vi "logForceActuatorInfo.vi"(8 "error in (no error)":errorcluster, 10 "EventForceActuatorInfo":T1, 11 "M1M3SAL in":refnum<class "M1M3SAL.lvclass">) -> (0 "error out":errorcluster, 3 "M1M3SAL out":refnum<class "M1M3SAL.lvclass">)   [LabVIEW 2016, in "M1M3SupportCommunicator.lvlib" / "M1M3SAL.lvclass"]
uses:
  M1M3SAL.lvclass
  DataTypes/Topics/EventForceActuatorInfo.ctl
  DataTypes/Topics/Parts/Timestamp.ctl
  DataTypes/MessageHeader.ctl
  DataTypes/MessageTypes.ctl
  DataTypes/MessageTopics.ctl
  M1M3SAL.lvclass/M1M3SAL.ctl
  writeU8.vi
  writeSGL.vi
  writeI64.vi
  writeBoolean.vi
  M1M3SupportCommunicator.lvlib
  DataTypes/Topics/M1M3SupportTopics.lvlib
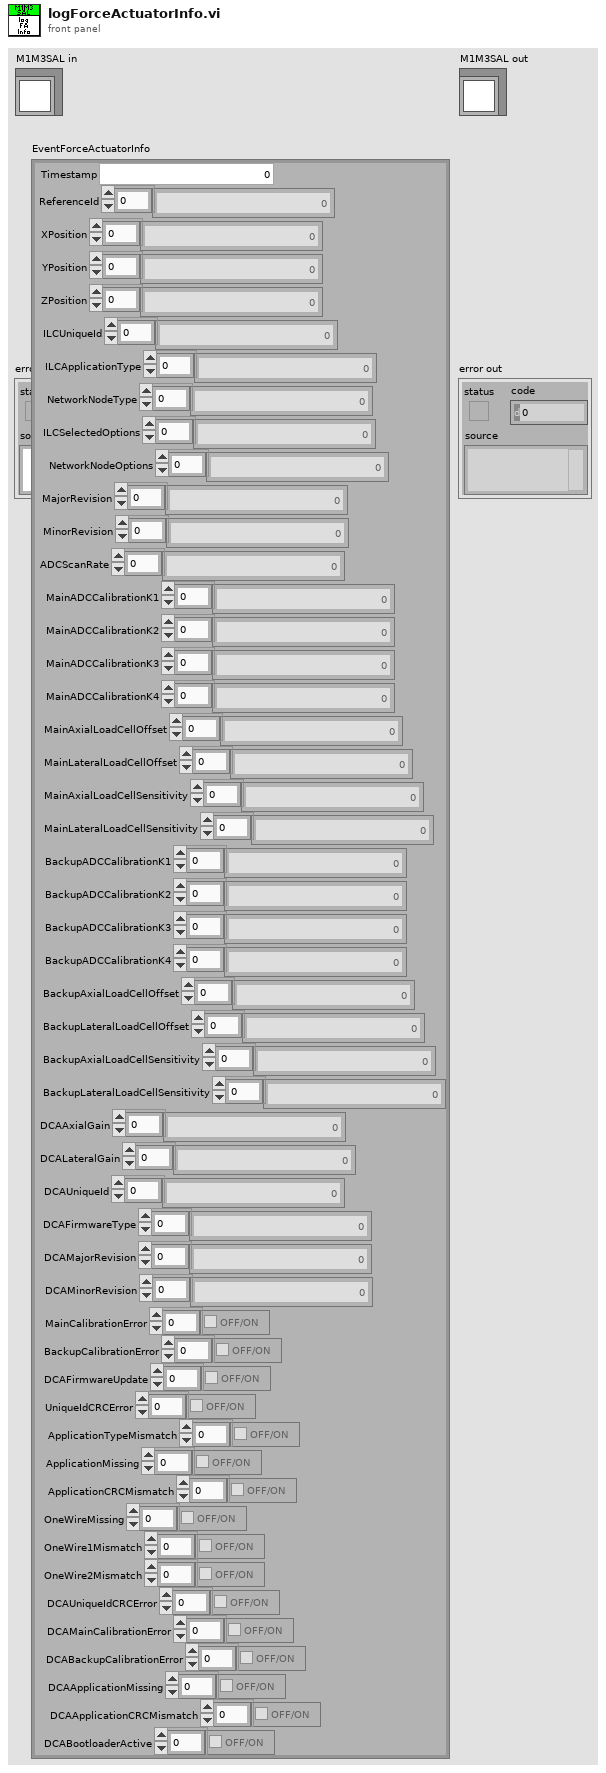
[diagram p1: front panel]
types:
  T1 = typedef "M1M3SupportTopics.lvlib/EventForceActuatorInfo.ctl" = cluster{"Timestamp":T2, "ReferenceId":i32[], "XPosition":sgl[], "YPosition":sgl[], "ZPosition":sgl[], "ILCUniqueId":i64[], "ILCApplicationType":u8[], "NetworkNodeType":u8[], "ILCSelectedOptions":u8[], "NetworkNodeOptions":u8[], "MajorRevision":u8[], "MinorRevision":u8[], "ADCScanRate":u8[], "MainADCCalibrationK1":sgl[], "MainADCCalibrationK2":sgl[], "MainADCCalibrationK3":sgl[], "MainADCCalibrationK4":sgl[], "MainAxialLoadCellOffset":sgl[], "MainLateralLoadCellOffset":sgl[], "MainAxialLoadCellSensitivity":sgl[], "MainLateralLoadCellSensitivity":sgl[], "BackupADCCalibrationK1":sgl[], "BackupADCCalibrationK2":sgl[], "BackupADCCalibrationK3":sgl[], "BackupADCCalibrationK4":sgl[], "BackupAxialLoadCellOffset":sgl[], "BackupLateralLoadCellOffset":sgl[], "BackupAxialLoadCellSensitivity":sgl[], "BackupLateralLoadCellSensitivity":sgl[], "DCAAxialGain":sgl[], "DCALateralGain":sgl[], "DCAUniqueId":i64[], "DCAFirmwareType":u8[], "DCAMajorRevision":u8[], "DCAMinorRevision":u8[], "MainCalibrationError":bool[], "BackupCalibrationError":bool[], "DCAFirmwareUpdate":bool[], "UniqueIdCRCError":bool[], "ApplicationTypeMismatch":bool[], "ApplicationMissing":bool[], "ApplicationCRCMismatch":bool[], "OneWireMissing":bool[], "OneWire1Mismatch":bool[], "OneWire2Mismatch":bool[], "DCAUniqueIdCRCError":bool[], "DCAMainCalibrationError":bool[], "DCABackupCalibrationError":bool[], "DCAApplicationMissing":bool[], "DCAApplicationCRCMismatch":bool[], "DCABootloaderActive":bool[]}
  T2 = typedef "M1M3SupportTopics.lvlib/Timestamp.ctl" = dbl
  T3 = typedef "M1M3SupportCommunicator.lvlib/MessageHeader.ctl" = cluster{"Type":T4, "Topic":T5, "Size":i32}
  T4 = typedef "M1M3SupportCommunicator.lvlib/MessageTypes.ctl" = enum8{"None", "PutSample", "GetNextSample", "LogEvent", "GetEvent", "IssueCommand", "CommandId", "WaitForCompletion", "AcceptCommand", "AckCommand"}
  T5 = typedef "M1M3SupportCommunicator.lvlib/MessageTopics.ctl" = enum8{"None", "ForceActuatorData", "MirrorForceData", "HardpointData", "AirData", "DynamicData", "FPGAData", "IMSData", "ForceActuatorStatus", "ElevationData", "HardpointStatus", "HardpointActuatorChase", "AirStatus", "ForceActuatorSafetyChecks", "ForceActuatorTest", "ActuatorBroadcastCounter", "StatusChecks", "CellChecks", "HardpointActuatorBreakaway", "RaiseMirrorComplete", "ILCCommunication", "ElevationAngleChecks", "DetailedState", "ServoLoops", "ForceActuatorInfo", "LowerMirrorComplete", "HardpointActuatorInfo", "SettingsApplied", "ErrorCode", "StartupChecks", "SummaryState", "SettingVersions", "ActuatorTestStatus", "AppliedSettingsMatchStart", "Enable", "EnterMaintenance", "Standby", "AbortLowerM1M3", "ApplyAberrationByForces", "ApplyAOSCorrectionByBendingModes", "ClearAOSCorrection", "Start", "RaiseM1M3", "TestForceActuator", "LowerM1M3", "ApplyAOSCorrectionByForces", "Disable", "ApplyAberationByBendingMode", "TestHardpoint", "ManipulateM1M3", "ClearAberration", "Exit", "TestAir", "AbortRaiseM1M3", "MoveHardpointActuators", "ExitMaintenance", "Shutdown"}
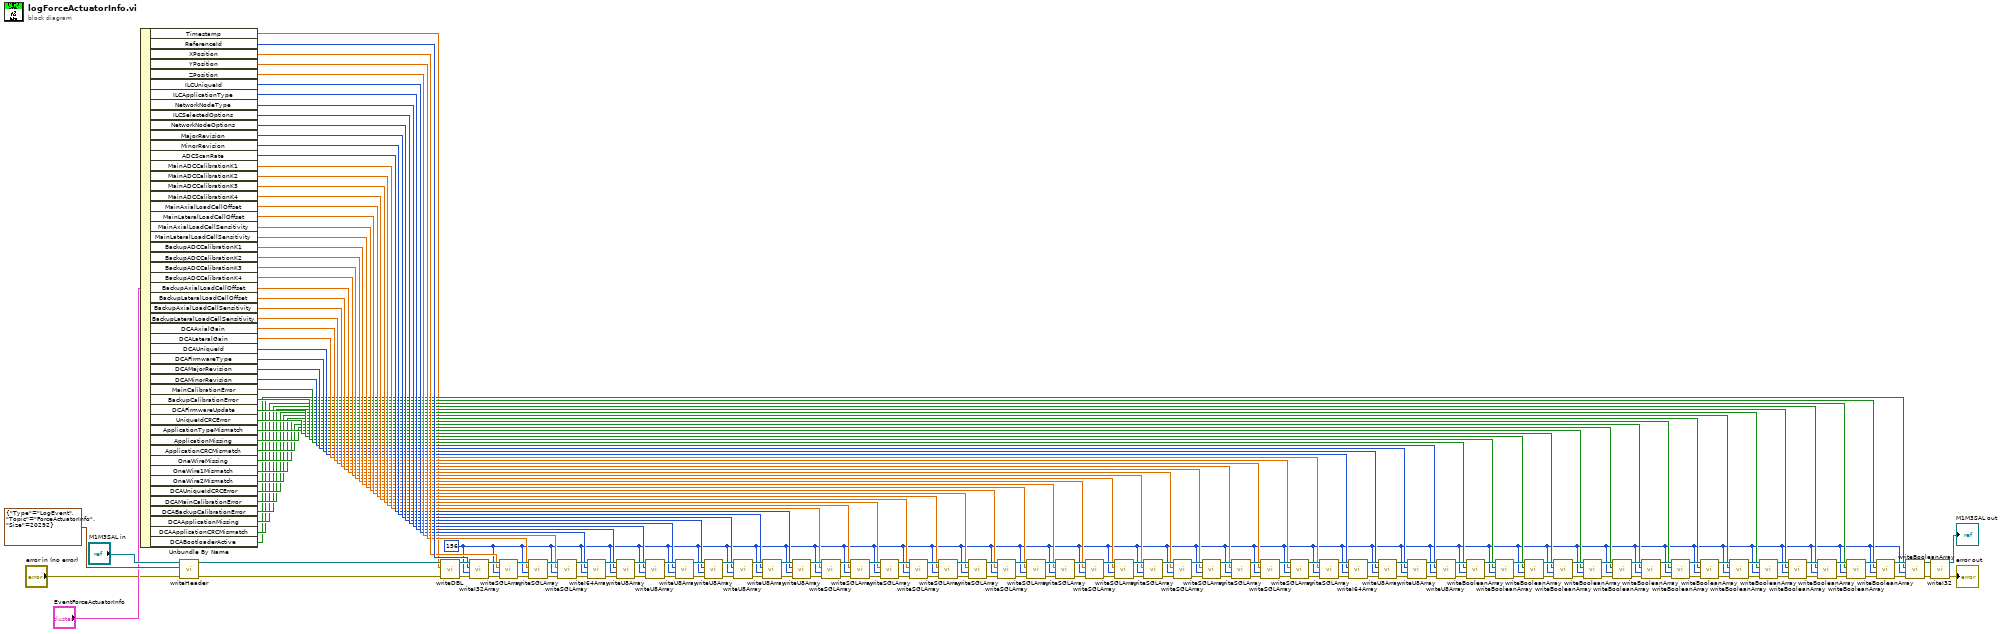
[diagram p0: block diagram]
diagram:
  w7 = 156
  n1 = Unbundle By Name("EventForceActuatorInfo") -> ("Timestamp"=w2:T2, "ReferenceId"=w155:i32[], "XPosition"=w154:sgl[], "YPosition"=w55:sgl[], "ZPosition"=w54:sgl[], "ILCUniqueId"=w53:i64[], "ILCApplicationType"=w52:u8[], "NetworkNodeType"=w51:u8[], "ILCSelectedOptions"=w50:u8[], "NetworkNodeOptions"=w49:u8[], "MajorRevision"=w48:u8[], "MinorRevision"=w47:u8[], "ADCScanRate"=w46:u8[], "MainADCCalibrationK1"=w45:sgl[], "MainADCCalibrationK2"=w44:sgl[], "MainADCCalibrationK3"=w43:sgl[], "MainADCCalibrationK4"=w42:sgl[], "MainAxialLoadCellOffset"=w41:sgl[], "MainLateralLoadCellOffset"=w40:sgl[], "MainAxialLoadCellSensitivity"=w39:sgl[], "MainLateralLoadCellSensitivity"=w38:sgl[], "BackupADCCalibrationK1"=w37:sgl[], "BackupADCCalibrationK2"=w36:sgl[], "BackupADCCalibrationK3"=w35:sgl[], "BackupADCCalibrationK4"=w34:sgl[], "BackupAxialLoadCellOffset"=w33:sgl[], "BackupLateralLoadCellOffset"=w32:sgl[], "BackupAxialLoadCellSensitivity"=w31:sgl[], "BackupLateralLoadCellSensitivity"=w30:sgl[], "DCAAxialGain"=w29:sgl[], "DCALateralGain"=w28:sgl[], "DCAUniqueId"=w27:i64[], "DCAFirmwareType"=w26:u8[], "DCAMajorRevision"=w25:u8[], "DCAMinorRevision"=w24:u8[], "MainCalibrationError"=w23:bool[], "BackupCalibrationError"=w22:bool[], "DCAFirmwareUpdate"=w21:bool[], "UniqueIdCRCError"=w20:bool[], "ApplicationTypeMismatch"=w19:bool[], "ApplicationMissing"=w18:bool[], "ApplicationCRCMismatch"=w17:bool[], "OneWireMissing"=w16:bool[], "OneWire1Mismatch"=w15:bool[], "OneWire2Mismatch"=w14:bool[], "DCAUniqueIdCRCError"=w13:bool[], "DCAMainCalibrationError"=w12:bool[], "DCABackupCalibrationError"=w11:bool[], "DCAApplicationMissing"=w10:bool[], "DCAApplicationCRCMismatch"=w9:bool[], "DCABootloaderActive"=w8:bool[])
  n2 = call "writeHeader.vi"("error in (no error)"="error in (no error)", "MessageHeader"=T3 {"Type"=enum."LogEvent", "Topic"=enum."ForceActuatorInfo", "Size"=20292}, "M1M3SAL in"="M1M3SAL in") -> ("error out"=w3:errorcluster, "M1M3SAL out"=w4:refnum<class "M1M3SAL.lvclass">)  [unwired: 7 in]
  n3 = call "writeDBL.vi"("error in (no error)"=w3, "Input"=w2, "M1M3SAL in"=w4) -> ("error out"=w158:errorcluster, "M1M3SAL out"=w159:refnum<class "M1M3SAL.lvclass">)  [unwired: 7 in]
  n4 = call "writeI32Array.vi"("error in (no error)"=w158, "Length"=w7, "Input"=w155, "M1M3SAL in"=w159) -> ("error out"=w156:errorcluster, "M1M3SAL out"=w157:refnum<class "M1M3SAL.lvclass">)  [unwired: 6 in]
  n5 = call "writeSGLArray.vi"("error in (no error)"=w156, "Length"=w7, "Input"=w154, "M1M3SAL in"=w157) -> ("error out"=w153:errorcluster, "M1M3SAL out"=w152:refnum<class "M1M3SAL.lvclass">)  [unwired: 6 in]
  n6 = call "writeSGLArray.vi"("error in (no error)"=w153, "Length"=w7, "Input"=w55, "M1M3SAL in"=w152) -> ("error out"=w151:errorcluster, "M1M3SAL out"=w150:refnum<class "M1M3SAL.lvclass">)  [unwired: 6 in]
  n7 = call "writeSGLArray.vi"("error in (no error)"=w151, "Length"=w7, "Input"=w54, "M1M3SAL in"=w150) -> ("error out"=w148:errorcluster, "M1M3SAL out"=w149:refnum<class "M1M3SAL.lvclass">)  [unwired: 6 in]
  n8 = call "writeI64Array.vi"("error in (no error)"=w148, "Length"=w7, "Input"=w53, "M1M3SAL in"=w149) -> ("error out"=w146:errorcluster, "M1M3SAL out"=w147:refnum<class "M1M3SAL.lvclass">)  [unwired: 6 in]
  n9 = call "writeU8Array.vi"("error in (no error)"=w146, "Length"=w7, "Input"=w52, "M1M3SAL in"=w147) -> ("error out"=w145:errorcluster, "M1M3SAL out"=w144:refnum<class "M1M3SAL.lvclass">)  [unwired: 6 in]
  n10 = call "writeU8Array.vi"("error in (no error)"=w145, "Length"=w7, "Input"=w51, "M1M3SAL in"=w144) -> ("error out"=w143:errorcluster, "M1M3SAL out"=w142:refnum<class "M1M3SAL.lvclass">)  [unwired: 6 in]
  n11 = call "writeU8Array.vi"("error in (no error)"=w143, "Length"=w7, "Input"=w50, "M1M3SAL in"=w142) -> ("error out"=w141:errorcluster, "M1M3SAL out"=w140:refnum<class "M1M3SAL.lvclass">)  [unwired: 6 in]
  n12 = call "writeU8Array.vi"("error in (no error)"=w141, "Length"=w7, "Input"=w49, "M1M3SAL in"=w140) -> ("error out"=w139:errorcluster, "M1M3SAL out"=w138:refnum<class "M1M3SAL.lvclass">)  [unwired: 6 in]
  n13 = call "writeU8Array.vi"("error in (no error)"=w139, "Length"=w7, "Input"=w48, "M1M3SAL in"=w138) -> ("error out"=w137:errorcluster, "M1M3SAL out"=w136:refnum<class "M1M3SAL.lvclass">)  [unwired: 6 in]
  n14 = call "writeU8Array.vi"("error in (no error)"=w137, "Length"=w7, "Input"=w47, "M1M3SAL in"=w136) -> ("error out"=w135:errorcluster, "M1M3SAL out"=w134:refnum<class "M1M3SAL.lvclass">)  [unwired: 6 in]
  n15 = call "writeU8Array.vi"("error in (no error)"=w135, "Length"=w7, "Input"=w46, "M1M3SAL in"=w134) -> ("error out"=w133:errorcluster, "M1M3SAL out"=w132:refnum<class "M1M3SAL.lvclass">)  [unwired: 6 in]
  n16 = call "writeSGLArray.vi"("error in (no error)"=w133, "Length"=w7, "Input"=w45, "M1M3SAL in"=w132) -> ("error out"=w131:errorcluster, "M1M3SAL out"=w130:refnum<class "M1M3SAL.lvclass">)  [unwired: 6 in]
  n17 = call "writeSGLArray.vi"("error in (no error)"=w131, "Length"=w7, "Input"=w44, "M1M3SAL in"=w130) -> ("error out"=w129:errorcluster, "M1M3SAL out"=w128:refnum<class "M1M3SAL.lvclass">)  [unwired: 6 in]
  n18 = call "writeSGLArray.vi"("error in (no error)"=w129, "Length"=w7, "Input"=w43, "M1M3SAL in"=w128) -> ("error out"=w127:errorcluster, "M1M3SAL out"=w126:refnum<class "M1M3SAL.lvclass">)  [unwired: 6 in]
  n19 = call "writeSGLArray.vi"("error in (no error)"=w127, "Length"=w7, "Input"=w42, "M1M3SAL in"=w126) -> ("error out"=w125:errorcluster, "M1M3SAL out"=w124:refnum<class "M1M3SAL.lvclass">)  [unwired: 6 in]
  n20 = call "writeSGLArray.vi"("error in (no error)"=w125, "Length"=w7, "Input"=w41, "M1M3SAL in"=w124) -> ("error out"=w123:errorcluster, "M1M3SAL out"=w122:refnum<class "M1M3SAL.lvclass">)  [unwired: 6 in]
  n21 = call "writeSGLArray.vi"("error in (no error)"=w123, "Length"=w7, "Input"=w40, "M1M3SAL in"=w122) -> ("error out"=w121:errorcluster, "M1M3SAL out"=w120:refnum<class "M1M3SAL.lvclass">)  [unwired: 6 in]
  n22 = call "writeSGLArray.vi"("error in (no error)"=w121, "Length"=w7, "Input"=w39, "M1M3SAL in"=w120) -> ("error out"=w119:errorcluster, "M1M3SAL out"=w118:refnum<class "M1M3SAL.lvclass">)  [unwired: 6 in]
  n23 = call "writeSGLArray.vi"("error in (no error)"=w119, "Length"=w7, "Input"=w38, "M1M3SAL in"=w118) -> ("error out"=w117:errorcluster, "M1M3SAL out"=w116:refnum<class "M1M3SAL.lvclass">)  [unwired: 6 in]
  n24 = call "writeSGLArray.vi"("error in (no error)"=w117, "Length"=w7, "Input"=w37, "M1M3SAL in"=w116) -> ("error out"=w115:errorcluster, "M1M3SAL out"=w114:refnum<class "M1M3SAL.lvclass">)  [unwired: 6 in]
  n25 = call "writeSGLArray.vi"("error in (no error)"=w115, "Length"=w7, "Input"=w36, "M1M3SAL in"=w114) -> ("error out"=w113:errorcluster, "M1M3SAL out"=w112:refnum<class "M1M3SAL.lvclass">)  [unwired: 6 in]
  n26 = call "writeSGLArray.vi"("error in (no error)"=w113, "Length"=w7, "Input"=w35, "M1M3SAL in"=w112) -> ("error out"=w111:errorcluster, "M1M3SAL out"=w110:refnum<class "M1M3SAL.lvclass">)  [unwired: 6 in]
  n27 = call "writeSGLArray.vi"("error in (no error)"=w111, "Length"=w7, "Input"=w34, "M1M3SAL in"=w110) -> ("error out"=w109:errorcluster, "M1M3SAL out"=w108:refnum<class "M1M3SAL.lvclass">)  [unwired: 6 in]
  n28 = call "writeSGLArray.vi"("error in (no error)"=w109, "Length"=w7, "Input"=w33, "M1M3SAL in"=w108) -> ("error out"=w107:errorcluster, "M1M3SAL out"=w106:refnum<class "M1M3SAL.lvclass">)  [unwired: 6 in]
  n29 = call "writeSGLArray.vi"("error in (no error)"=w107, "Length"=w7, "Input"=w32, "M1M3SAL in"=w106) -> ("error out"=w105:errorcluster, "M1M3SAL out"=w104:refnum<class "M1M3SAL.lvclass">)  [unwired: 6 in]
  n30 = call "writeSGLArray.vi"("error in (no error)"=w105, "Length"=w7, "Input"=w31, "M1M3SAL in"=w104) -> ("error out"=w103:errorcluster, "M1M3SAL out"=w102:refnum<class "M1M3SAL.lvclass">)  [unwired: 6 in]
  n31 = call "writeSGLArray.vi"("error in (no error)"=w103, "Length"=w7, "Input"=w30, "M1M3SAL in"=w102) -> ("error out"=w101:errorcluster, "M1M3SAL out"=w100:refnum<class "M1M3SAL.lvclass">)  [unwired: 6 in]
  n32 = call "writeSGLArray.vi"("error in (no error)"=w101, "Length"=w7, "Input"=w29, "M1M3SAL in"=w100) -> ("error out"=w99:errorcluster, "M1M3SAL out"=w98:refnum<class "M1M3SAL.lvclass">)  [unwired: 6 in]
  n33 = call "writeSGLArray.vi"("error in (no error)"=w99, "Length"=w7, "Input"=w28, "M1M3SAL in"=w98) -> ("error out"=w96:errorcluster, "M1M3SAL out"=w97:refnum<class "M1M3SAL.lvclass">)  [unwired: 6 in]
  n34 = call "writeI64Array.vi"("error in (no error)"=w96, "Length"=w7, "Input"=w27, "M1M3SAL in"=w97) -> ("error out"=w94:errorcluster, "M1M3SAL out"=w95:refnum<class "M1M3SAL.lvclass">)  [unwired: 6 in]
  n35 = call "writeU8Array.vi"("error in (no error)"=w94, "Length"=w7, "Input"=w26, "M1M3SAL in"=w95) -> ("error out"=w93:errorcluster, "M1M3SAL out"=w92:refnum<class "M1M3SAL.lvclass">)  [unwired: 6 in]
  n36 = call "writeU8Array.vi"("error in (no error)"=w93, "Length"=w7, "Input"=w25, "M1M3SAL in"=w92) -> ("error out"=w91:errorcluster, "M1M3SAL out"=w90:refnum<class "M1M3SAL.lvclass">)  [unwired: 6 in]
  n37 = call "writeU8Array.vi"("error in (no error)"=w91, "Length"=w7, "Input"=w24, "M1M3SAL in"=w90) -> ("error out"=w89:errorcluster, "M1M3SAL out"=w88:refnum<class "M1M3SAL.lvclass">)  [unwired: 6 in]
  n38 = call "writeBooleanArray.vi"("error in (no error)"=w89, "Length"=w7, "Input"=w23, "M1M3SAL in"=w88) -> ("error out"=w87:errorcluster, "M1M3SAL out"=w86:refnum<class "M1M3SAL.lvclass">)  [unwired: 6 in]
  n39 = call "writeBooleanArray.vi"("error in (no error)"=w87, "Length"=w7, "Input"=w22, "M1M3SAL in"=w86) -> ("error out"=w85:errorcluster, "M1M3SAL out"=w84:refnum<class "M1M3SAL.lvclass">)  [unwired: 6 in]
  n40 = call "writeBooleanArray.vi"("error in (no error)"=w85, "Length"=w7, "Input"=w21, "M1M3SAL in"=w84) -> ("error out"=w83:errorcluster, "M1M3SAL out"=w82:refnum<class "M1M3SAL.lvclass">)  [unwired: 6 in]
  n41 = call "writeBooleanArray.vi"("error in (no error)"=w83, "Length"=w7, "Input"=w20, "M1M3SAL in"=w82) -> ("error out"=w81:errorcluster, "M1M3SAL out"=w80:refnum<class "M1M3SAL.lvclass">)  [unwired: 6 in]
  n42 = call "writeBooleanArray.vi"("error in (no error)"=w81, "Length"=w7, "Input"=w19, "M1M3SAL in"=w80) -> ("error out"=w79:errorcluster, "M1M3SAL out"=w78:refnum<class "M1M3SAL.lvclass">)  [unwired: 6 in]
  n43 = call "writeBooleanArray.vi"("error in (no error)"=w79, "Length"=w7, "Input"=w18, "M1M3SAL in"=w78) -> ("error out"=w77:errorcluster, "M1M3SAL out"=w76:refnum<class "M1M3SAL.lvclass">)  [unwired: 6 in]
  n44 = call "writeBooleanArray.vi"("error in (no error)"=w77, "Length"=w7, "Input"=w17, "M1M3SAL in"=w76) -> ("error out"=w75:errorcluster, "M1M3SAL out"=w74:refnum<class "M1M3SAL.lvclass">)  [unwired: 6 in]
  n45 = call "writeBooleanArray.vi"("error in (no error)"=w75, "Length"=w7, "Input"=w16, "M1M3SAL in"=w74) -> ("error out"=w73:errorcluster, "M1M3SAL out"=w72:refnum<class "M1M3SAL.lvclass">)  [unwired: 6 in]
  n46 = call "writeBooleanArray.vi"("error in (no error)"=w73, "Length"=w7, "Input"=w15, "M1M3SAL in"=w72) -> ("error out"=w71:errorcluster, "M1M3SAL out"=w70:refnum<class "M1M3SAL.lvclass">)  [unwired: 6 in]
  n47 = call "writeBooleanArray.vi"("error in (no error)"=w71, "Length"=w7, "Input"=w14, "M1M3SAL in"=w70) -> ("error out"=w69:errorcluster, "M1M3SAL out"=w68:refnum<class "M1M3SAL.lvclass">)  [unwired: 6 in]
  n48 = call "writeBooleanArray.vi"("error in (no error)"=w69, "Length"=w7, "Input"=w13, "M1M3SAL in"=w68) -> ("error out"=w67:errorcluster, "M1M3SAL out"=w66:refnum<class "M1M3SAL.lvclass">)  [unwired: 6 in]
  n49 = call "writeBooleanArray.vi"("error in (no error)"=w67, "Length"=w7, "Input"=w12, "M1M3SAL in"=w66) -> ("error out"=w65:errorcluster, "M1M3SAL out"=w64:refnum<class "M1M3SAL.lvclass">)  [unwired: 6 in]
  n50 = call "writeBooleanArray.vi"("error in (no error)"=w65, "Length"=w7, "Input"=w11, "M1M3SAL in"=w64) -> ("error out"=w63:errorcluster, "M1M3SAL out"=w62:refnum<class "M1M3SAL.lvclass">)  [unwired: 6 in]
  n51 = call "writeBooleanArray.vi"("error in (no error)"=w63, "Length"=w7, "Input"=w10, "M1M3SAL in"=w62) -> ("error out"=w61:errorcluster, "M1M3SAL out"=w60:refnum<class "M1M3SAL.lvclass">)  [unwired: 6 in]
  n52 = call "writeBooleanArray.vi"("error in (no error)"=w61, "Length"=w7, "Input"=w9, "M1M3SAL in"=w60) -> ("error out"=w59:errorcluster, "M1M3SAL out"=w58:refnum<class "M1M3SAL.lvclass">)  [unwired: 6 in]
  n53 = call "writeBooleanArray.vi"("error in (no error)"=w59, "Length"=w7, "Input"=w8, "M1M3SAL in"=w58) -> ("error out"=w56:errorcluster, "M1M3SAL out"=w57:refnum<class "M1M3SAL.lvclass">)  [unwired: 6 in]
  n54 = call "writeI32.vi"("error in (no error)"=w56, "M1M3SAL in"=w57) -> ("error out"=→"error out":errorcluster, "M1M3SAL out"=→"M1M3SAL out":refnum<class "M1M3SAL.lvclass">)  [unwired: 8 in]
